vi "FestoCPX.Station.LaserPress.Move.vi"(8 "error in":errorcluster, 10 "Position":T1) -> (0 "error out":errorcluster)   [LabVIEW 2015]
uses:
  tools/EventLog/EventLog.EventSource.ctl
  tools/Translator/Translator.Message.ctl
  FestoCPX.DI.Signal.ctl
  FestoCPX.DO.Signal.ctl
  FestoCPX.Valve(2out2in).vi
  tools/EventLog/EventLog.CreateError(array).vi
  Station/Station.ValvePosition.ctl
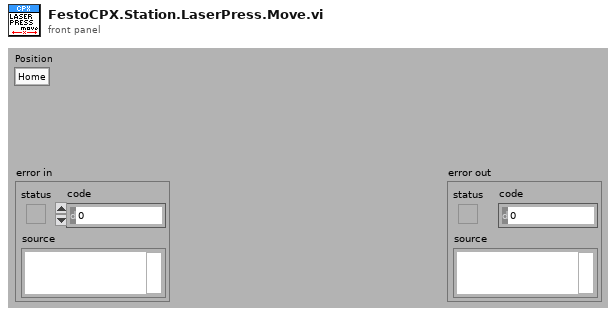
[diagram p1: front panel]
types:
  T1 = typedef "Station.ValvePosition.ctl" = enum16{"Home", "Work"}
  T2 = typedef "Translator.Message.ctl" = enum16{"-", "Event confirmed", "Log out", "Log in", "Shutdown", "Cancel", "Start", "On", "Off", "OK", "NOK", "NOK %s", "Home", "Work", "In progress...", "Missing", "Empty", "Hardware failure", "Initial", "Error %d >> %s", "Error %d >> %s >> %s", "Msg %d >> %s", "Unable to reset Laser Interlock", "Unable to reset Laser Shutterlock. Laser not ready", "Starting %s", "Quitting %s", "Configured", "Initializing", "Quitting", "Loading", "Running", "Stopped", "Summary", "Laser", "Do you want to continue?", "Station is not based. Do you want to exit?", "Station requires changeover. Do you want to run the test?", "Test options are not set as default. Do you want to continue?", "Connect ATEQ to terminal and set leakage to 0", "Set no leakage at ATEQ", "Set desired leakage at ATEQ at terminal M1 or skip", "Set desired leakage at ATEQ at terminal M3/M21/M22 or skip", "Set desired leakage at ATEQ at terminal M12 or skip", "Set desired leakage at ATEQ at terminal M1/M3 or skip", "Set desired leakage at ATEQ at terminal M21/M22 or skip", "Set desired leakage at ATEQ at terminal M1/M21/M22 or skip", "Calibration", "Log out?", "System", "All", "IDLE", "Translating...%s", "Not found", "Alarm %s", "Run", "Skip", "Abort", "Repeat", "Please wait...", "Database disconnected", "Database disconnected - changeover disabled!", "Login to database successful", "Login to database failed: %d; %s", "Unable to check the product status of reference %d - database disconnected", "Unable to set the product status of reference %d - database disconnected", "Variant file backup %s", "Read steps (%s)", "Result", "Station armed!", "Station requires changeover!", "Select reference number...", "EMERGENCY CURTAIN", "EMERGENCY BUTTON - press Control button", "EMERGENCY DOOR - press Control button", "Unable to reset safety circuit - Emergency Button pressed", "Unable to reset safety circuit - Emergency Doors open", "Station not based", "Station basing...", "Unkown reference", "Reference %d missing", "Test %s", "Test OK", "Test NOK", "Test NOK - press Confirm button", "Test error - press Confirm button", "Test stopped", "Station ready / Prepare product", "Station ready / Press start to scan product", "Station ready / Scanning product", "Rotating table...", "Rotating table... on hold by curtain", "Table rotated in %.1f seconds", "Table rotation aborted - Emergency button", "Table rotation aborted - Emergency door", "Table rotation aborted - Air pressure 1 off", "Table rotation aborted - Air pressure 2 off", "Test running... / Prepare next product", "Test running... / Press start to scan next product", "Test running... / Scanning next product...", "Test running... / Next products will start automatically", "Test running... / Scanning failed", "Stopping test...", "Finalizing test...", "Sequence folder '%s' is missing", "File '%s' is missing", "File '%s' is broken", "File '%s' is running", "Log file '%s' started", "Step '%s' added to log file", "Step '%s' graph added to log file", "Log file '%s' ended", "Log file '%s' ignored", "Log file '%s' exported", "Log file '%s' export failed", "Wrong serial number in log file", "Test steps are missing", "Output %s = %.3f", "Unable to output %s = %.1f (FB = %.1f; SP = %.1f)", "Unable to stabilize %s = %.1f (SP = %.1f)", "Assembly timeout", "Disassembly timeout", "Assembly %d | %25s | %.02f | %d", "Disassembly %d | %25s | %.02f | %d", "Process param '%s' not found in DB", "Process param '%s' wrong order", "Process param '%s' value %.3f out of limits (%.3f; %.3f)", "Step%d param '%s' not found in DB", "Step%d param '%s' wrong order", "Step%d param '%s' value %.3f out of limits (%.3f; %.3f)", "Step%d EV '%s' not found in DB", "Step%d EV '%s' wrong order", "Reference %d accepted", "Sequence started", "Sequence done", "Sequence aborted at step %d", "Sequence aborted at work", "Sequence aborted at home", "Sequence stopped at step %d", "Sequence error at step %d", "Seqeunce error at home", "Sequence error at work", "Scan plate failed", "Scan laser failed", "Scan plate failed. Error %s", "Scan laser failed. Error %s", "Scan plate failed. Scanner disconnected", "Scan laser failed. Scanner disconnected", "Scan plate failed. Wrong reference %d (expected %d)", "Scan plate failed. Serial number %d/%d did not pass the previous station (status %d)", "Scan plate OK %d/%d", "Scan laser OK", "Scan plate failed. Code missing", "Scan laser failed. Code missing", "Plate scanner OK", "Plate scanner failed. Press confirm button", "Scanning plate...", "%s = %d", "%s = %d->%d", "Motor initialized", "Motor homing", "Motor homed", "Motor home timeout", "Motor home failure. Unable to reset encoder counter (motor pos %.2f; enc pos %.2f)", "Motor started @ %.2f (%s; %.2f; %.1f)", "Motor updated @ %.2f (%s; %.2f; %.1f)", "Motor stopped @ %.2f", "Motor stop timeout", "Motor reached the position @ %.2f", "Motor reached the torque @ %.2f; %.2f", "Motor reached the pressure @ %.2f; %.2f", "Motor timeout (sp %.2f; pv %.2f)", "Unable to move motor - Forks not in Home position", "Screwdriver start timeout", "Screwdriver stop timeout", "Not homed", "Leak test timeout", "Unable to set %s = %.2f - air pressure off", "Unable to reset Emergency Circuit - emg button", "Unable to reset Emergency Circuit - light curtain", "Unable to reset Emergency Circuit - door open", "Unable to set digital output '%s' = %d", "Unable to switch on Air Main Valve - timeout", "Unable to switch off Air Main Valve - timeout", "Unable to rotate Table - timeout", "Unable to rotate Table - air pressure off", "Unable to rotate Table - Press not in Home position", "Unable to rotate Table - Pneumatic & Electric Conn not in Home position", "Unable to rotate Table - Exhaust Conn not in Home position", "Unable to rotate Table - unlock before movement timeout", "Unable to rotate Table - lock after movement timeout", "Unable to move Table Lock to %s position - timeout", "Unable to move Table Lock to %s position - air pressure off", "Unable to move Table Lock to %s position - Table not in position", "Unable to move Product Press to %s position - timeout", "Unable to move Product Press to %s position - air pressure off", "Unable to move Product Press to %s position - Table not locked", "Unable to move Product Press to %s position - Pneumatic & Electric Conn not in Home position", "Unable to move Product Press to %s position - Exhaust Conn not in Home position", "Unable to move Pneumatic & Electric Conn to %s position - timeout", "Unable to move Pneumatic & Electric Conn to %s position - air pressure off", "Unable to move Pneumatic & Electric Conn to %s position - Product Press not in Work position", "Unable to move Vent %s to %s position - timeout", "Unable to move Vent %s to %s position - air pressure off", "Unable to move Vent %s to %s position - Product Press not in Work position", "Unable to move Laser Press to %s position - timeout", "Unable to move Laser Press to %s position - air pressure off", "Unable to move Laser Press to %s position - Table not locked"}
  T3 = typedef "EventLog.EventSource.ctl" = enum16{"All", "Gui", "Ref", "File", "Seq", "Scan", "Lock", "AO", "AI", "CI", "DIO", "CPX", "PS", "Proda", "Trace", "Laser", "Keyence"}
  T4 = typedef "FestoCPX.DO.Signal.ctl" = enum16{"Start Button LED", "White Button LED", "Blue Button LED", "Red Button LED", "Safety Circuit Reset", "Air Main Valve", "Laser Interlock", "Laser Shutterlock", "Traffic Light Red", "Traffic Light Orange", "Traffic Light Green", "Horn", "Q1 Vent B Work", "Q1 Vent B Home", "Q2 Vent A Work", "Q2 Vent A Home", "Q3 Product Press A Work", "Q3 Product Press A Home", "Q4 Product Press B Work", "Q4 Product Press B Home", "Q5 Pneumatic Connection A Work", "Q5 Pneumatic Connection A Home", "Q6 Pneumatic Connection B Work", "Q6 Pneumatic Connection B Home", "Q7 Laser Press Work", "Q7 Laser Press Home", "Q8 Table Lock Work", "Q8 Table Lock Home", "Q13 Table Turn Work", "Q13 Table Turn Home"}
  T5 = typedef "FestoCPX.DI.Signal.ctl" = enum16{"S.C. Emergency Stop", "S.C. Light Curtain", "S.C. Doors", "S.C. Table Turn", "Air Pressure 1", "Air Pressure 2", "Start Button", "White Button", "Blue Button", "Red Button", "Product present landing A", "Product present landing B", "Product present unloading A", "Product present unloading B", "Pneumatic conection's add A", "Pneumatic conection's add B", "Vent B Work", "Vent B Home", "Vent A Work", "Vent A Home", "Lock Table", "Product Press A Work", "Product Press A Home", "Product Press B Work", "Product Press B Home", "Pneumatic Connection A Work", "Pneumatic Connection A Home", "Pneumatic Connection B Work", "Pneumatic Connection B Home", "Laser Press Work", "Laser Press Home"}
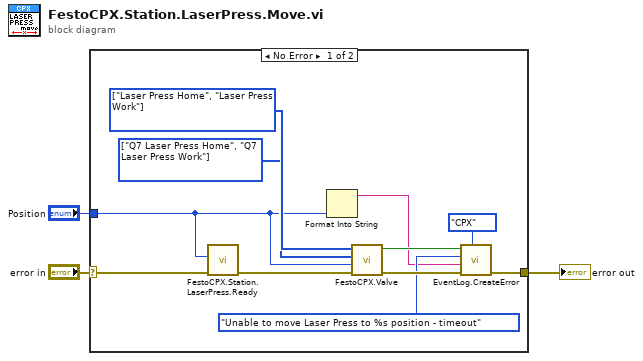
[diagram p0: block diagram]
diagram:
  n1 = case shown="No Error" "error in" {
    selector: "error in" -> [w12 w15]
    tunnel: [w14 w15] -> w3
    tunnel: "Position" -> [w5 _]
    frame No Error {
      w6 = T4[] [enum."Q7 Laser Press Home", enum."Q7 Laser Press Work"] items=["Start Button LED", "White Button LED", "Blue Button LED", "Red Button LED", "Safety Circuit Reset", "Air Main Valve", "Laser Interlock", "Laser Shutterlock", "Traffic Light Red", "Traffic Light Orange", "Traffic Light Green", "Horn", "Q1 Vent B Work", "Q1 Vent B Home", "Q2 Vent A Work", "Q2 Vent A Home", "Q3 Product Press A Work", "Q3 Product Press A Home", "Q4 Product Press B Work", "Q4 Product Press B Home", "Q5 Pneumatic Connection A Work", "Q5 Pneumatic Connection A Home", "Q6 Pneumatic Connection B Work", "Q6 Pneumatic Connection B Home", "Q7 Laser Press Work", "Q7 Laser Press Home", "Q8 Table Lock Work", "Q8 Table Lock Home", "Q13 Table Turn Work", "Q13 Table Turn Home"]
      w7 = T5[] [enum."Laser Press Home", enum."Laser Press Work"] items=["S.C. Emergency Stop", "S.C. Light Curtain", "S.C. Doors", "S.C. Table Turn", "Air Pressure 1", "Air Pressure 2", "Start Button", "White Button", "Blue Button", "Red Button", "Product present landing A", "Product present landing B", "Product present unloading A", "Product present unloading B", "Pneumatic conection's add A", "Pneumatic conection's add B", "Vent B Work", "Vent B Home", "Vent A Work", "Vent A Home", "Lock Table", "Product Press A Work", "Product Press A Home", "Product Press B Work", "Product Press B Home", "Pneumatic Connection A Work", "Pneumatic Connection A Home", "Pneumatic Connection B Work", "Pneumatic Connection B Home", "Laser Press Work", "Laser Press Home"]
      n2 = call "FestoCPX.Station.LaserPress.Ready.vi"("error in"=w12, "Position"=w5) -> ("error out"=w10:errorcluster)  [unwired: 8 in, 1 out]
      n3 = Format Into String(w5) -> (resulting string=w4:string)  [unwired: 3 in, 1 out]
      n4 = call-poly "FestoCPX.Valve.vi"("error in (no error)"=w10, "Position"=w5, "Valve outputs"=w6, "Inputs"=w7) -> ("error out"=w13:errorcluster, "Timeout?"=w11:bool)  [unwired: 6 in]
      n5 = call-poly "EventLog.CreateError.vi"("Source (All)"=EventLog.EventSource."CPX", "error in"=w13, "args"=w4, "msg"=Translator.Message."Unable to move Laser Press to %s position - timeout", "create (T)"=w11) -> ("error out"=w14:errorcluster)  [unwired: 5 in, 1 out]
    }
    frame Error {
    }
  }
  "error out" <- w3
